vi "Get All Input Parameters.vi"(8 "error in (no error)":errorcluster, 11 "Parametric VI Call In":refnum<class "Parametric VI Call.lvclass">) -> (0 "error out":errorcluster, 2 "Input Parameters":map{string, variant}(c390))   [LabVIEW 2020, in "Parametric VI Call.lvclass"]
uses:
  Parametric VI Call.lvclass
  Parametric VI Call.lvclass/Parametric VI Call.ctl
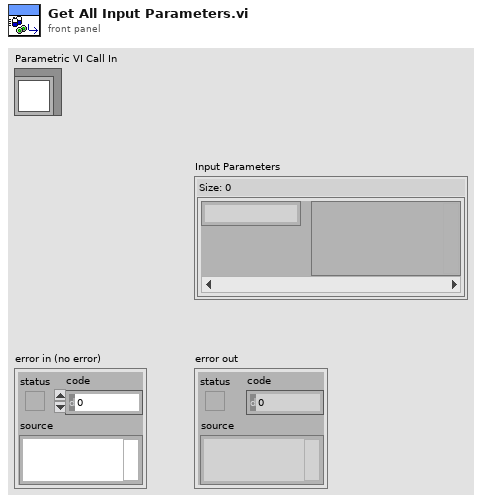
[diagram p1: front panel]
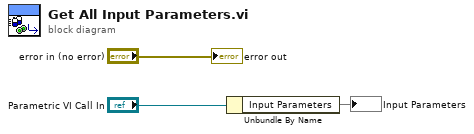
[diagram p0: block diagram]
diagram:
  n1 = Unbundle By Name("Parametric VI Call In") -> ("Input Parameters"=→"Input Parameters":map{string, variant})
  "error out" <- "error in (no error)"
